vi "Scripter Cleanup.vi"(8 "error in (no error)":errorcluster, 11 "Coupled Message Rescripter in":refnum<class "Message Scripter.lvclass">) -> (0 "error out":errorcluster)   [LabVIEW 2020, in "Message Rescripter.lvlib"]
uses:
  Message Rescripter.lvlib
  MessageMakerProvider/_Message Maker/_Maker Classes/Message Scripter/Message Scripter.lvclass
  <vilib>/Utility/EditLVLibs/Edit LVLibs.lvlib
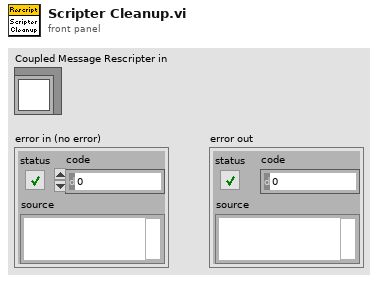
[diagram p1: front panel]
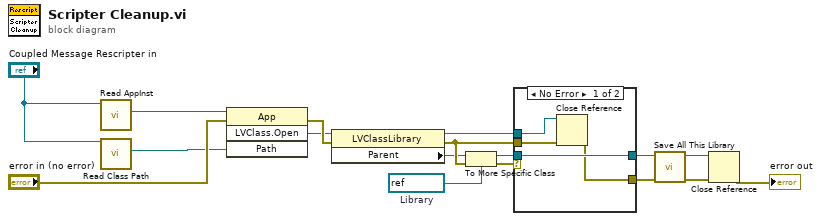
[diagram p0: block diagram]
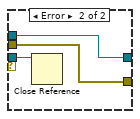
[diagram p2: hidden frame]
diagram:
  w8 = refnum<vi> refnum  # Library
  n1 = call "Read AppInst.vi"("Message Maker in"="Coupled Message Rescripter in") -> ("AppInst"=w2:refnum<vi>)  [unwired: 10 in]
  n2 = call "Read Class Path.vi"("Message Scripter in"="Coupled Message Rescripter in") -> ("Class Path"=w3:path)  [unwired: 10 in]
  n3 = invoke class="App" method="LVClass.Open"(reference=w2, error in="error in (no error)", "Path"=w3) -> (error out=w17:errorcluster, "LVClass.Open"=w6:refnum<vi>)  [unwired: 1 in, 2 out]
  n4 = property class="LVClassLibrary"(reference=w6, error in=w17) -> (reference out=w12:refnum<vi>, error out=w10:errorcluster, "Parent"=w7:refnum<vi>)
  n5 = To More Specific Class(target class=w8, reference=w7, error in=w10) -> (specific class reference=w11:refnum<vi>, error out=w9:errorcluster)
  n6 = case shown="No Error" w9 {
    tunnel: w10 -> [w20 w22]
    tunnel: w11 -> [w21 w24]
    tunnel: [w21 w23] -> w13
    tunnel: w12 -> [w19 w23]
    tunnel: [w18 w22] -> w16
    frame No Error {
      n7 = Close Reference(reference=w19, error in (no error)=w20) -> (error out=w18:errorcluster)
    }
    frame Error {
      n8 = Close Reference(reference=w24) -> ()  [unwired: 1 in, 1 out]
    }
  }
  n9 = call <vilib>:"Save All This Library.vi"("error in (no error)"=w16, "Library in"=w13) -> ("error out"=w15:errorcluster, "Library out"=w14:refnum<vi>)  [unwired: 8 in]
  n10 = Close Reference(reference=w14, error in (no error)=w15) -> (error out=→"error out":errorcluster)
